vi "Get JSON Data.vi"(6 "Force Hide":bool, 7 "Evaluate Pane Move":bool, 8 "error in (no error)":errorcluster, 9 "Force Get All Data":bool, 10 "VI Reference":refnum<vi>, 11 "Object In":refnum<class "Object.lvclass">) -> (0 "error out":errorcluster, 2 "JSON string":string, 3 "Object Out":refnum<class "Object.lvclass">)   [LabVIEW 2017, in "Front Panel Publisher.lvlib" / "Object.lvclass"]
uses:
  Object.lvclass
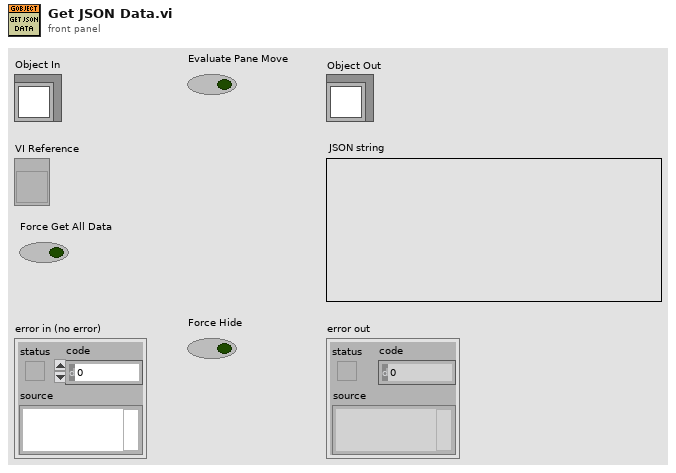
[diagram p1: front panel]
types:
  T1 = typedef "Front Panel Publisher.lvlib/Object.lvclass/Attributes.ctl" = cluster{"UID":i32, "Type":string, "Starting Location":T2, "Reference":refnum<vi>, "Cluster Component":bool, "Starting Rect Position":cluster{"Left":i16, "Top":i16}, "Owning Pane":refnum<vi>, "Master Total Rect Delta":T3}
  T2 = typedef "Front Panel Publisher.lvlib/Object.lvclass/Coordinates.ctl" = cluster{"Left":i32, "Top":i32, "Height":u32, "Width":u32}
  T3 = typedef "LVRectTypeDef.ctl" = cluster{"Left":i16, "Top":i16, "Right":i16, "Bottom":i16}
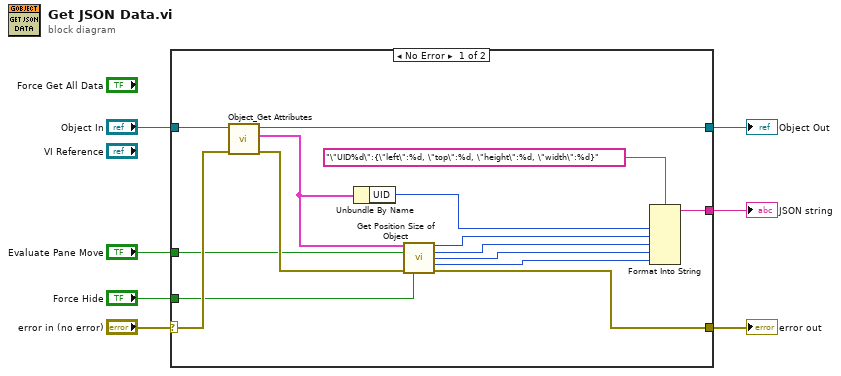
[diagram p0: block diagram]
diagram:
  n1 = case shown="No Error" "error in (no error)" {
    selector: "error in (no error)" -> [w22 w24]
    tunnel: [w12 w24] -> w6
    tunnel: [w20 w23] -> w4
    tunnel: "Object In" -> [w21 w23]
    tunnel: [w11 _] -> w3
    tunnel: "Evaluate Pane Move" -> [w10 _]
    tunnel: "Force Hide" -> [w9 _]
    frame No Error {
      n2 = call "Object_Get Attributes.vi"("error in (no error)"=w22, "Object In"=w21) -> ("error out"=w13:errorcluster, "Object Attributes"=w8:T1, "Object Out"=w20:refnum<class "Object.lvclass">)  [unwired: 7 in]
      n3 = Unbundle By Name(w8) -> ("UID"=w18:i32)
      n4 = call "Get Position Size of Object.vi"("Object Attributes"=w8, "Evaluate Pane Move"=w10, "error in (no error)"=w13, "Force Hide"=w9) -> ("Left"=w17:i32, "Top"=w16:i32, "Height"=w15:u32, "Width"=w14:u32, "error out"=w12:errorcluster)  [unwired: 6 in, 1 out]
      n5 = Format Into String(format string="\"UID%d\":{\"left\":%d, \"top\":%d, \"height\":%d, \"width\":%d}", w18, w17, w16, w15, w14) -> (resulting string=w11:string)  [unwired: 2 in, 1 out]
    }
    frame Error {
    }
  }
  "error out" <- w6
  "Object Out" <- w4
  "JSON string" <- w3
